vi "Monitor External Variable Clock.vi"() -> ()   [LabVIEW 2026]
uses:
  <vilib>/DAQmx/read.llb/DAQmx Read (Analog 1D Wfm NChan NSamp).vi
  <vilib>/FPGAPlugInAG/PXIe-7856R/niLvFpga_Open_PXIe-7856R.vi
  <vilib>/rvi/interface/common/dynamic/niFpgaDynamicAddResources.vi
  <vilib>/Utility/error.llb/Error Cluster From Error Code.vi
  <vilib>/rvi/errors/niLvFpgaAdjustHostInterfaceError.vi
  <vilib>/FPGAPlugInAG/Dynamic/niLvFpga_Run_Dynamic.vi
  <vilib>/DAQmx/create/channels.llb/DAQmx Create Channel (AI-Voltage-Basic).vi
  <vilib>/DAQmx/configure/timing.llb/DAQmx Timing (Sample Clock).vi
  <vilib>/DAQmx/miscellaneous.llb/DAQmx Fill In Error Info.vi
  <vilib>/measure/mascope.llb/Pulse Measurements N chan.vi
  <vilib>/FPGAPlugInAG/Dynamic/niLvFpga_Close_Dynamic.vi
  <vilib>/rvi/interface/nirviOpenFPGA/nirviOpenFPGA.xnode
  FPGA Bitfiles/PulseAndClockGeneration.lvbitx
  FPGA/Pulse and Clock Generation.vi
  <vilib>/rvi/interface/nirviReadWriteControl/nirviReadWriteControl.xnode
  <vilib>/rvi/interface/nirviMethod/nirviMethod.xnode
  <vilib>/rvi/interface/nirviCloseFPGA/nirviCloseFPGA.xnode
  <vilib>/rvi/interface/Simulation/niFpgaSimulationCallBeginRW.vi
  NiFpgaLv.dll
  <vilib>/measure/NI_MAPro.lvlib
panel:
  out "Frequency Hz":dbl
  in  "stop":bool
  out "Waveform Graph":waveform(dbl)[](graph)
  out "error out":errorcluster
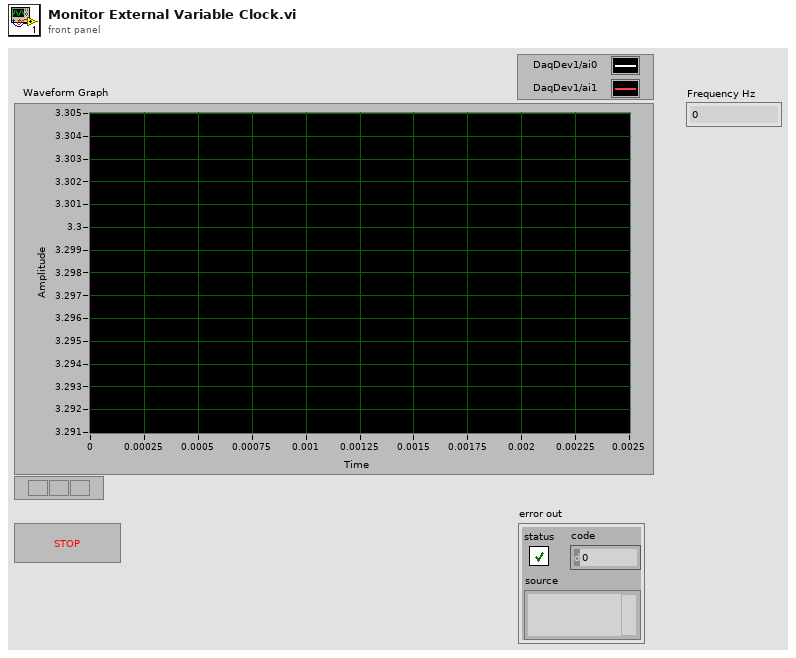
[diagram p1: front panel]
types:
  T1 = cluster{"high ref level":dbl, "mid ref level":dbl, "low ref level":dbl, "ref units":u16}
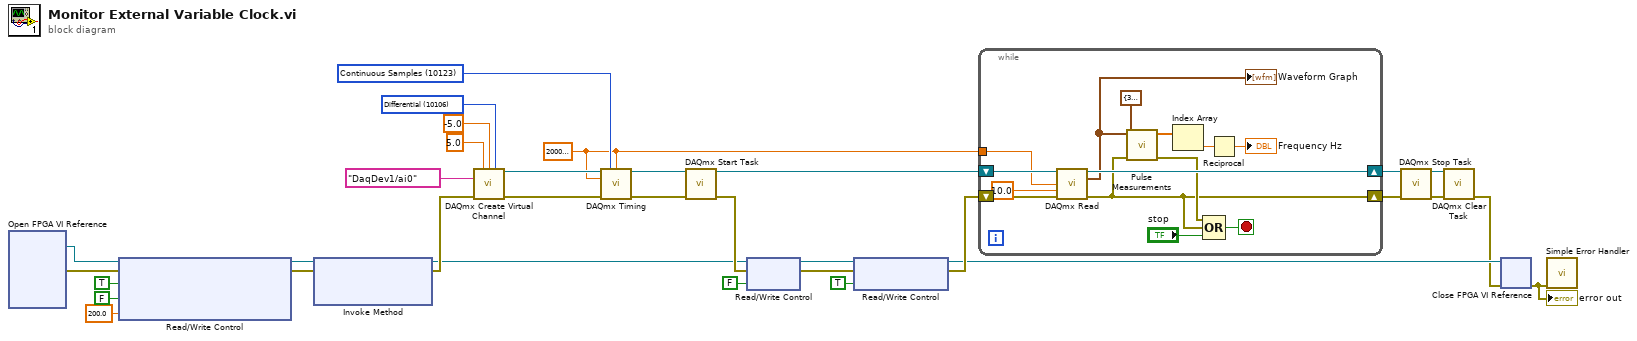
[diagram p0: block diagram]
diagram:
  w2 = 2000000.0 ("rate")
  w27 = 10123 items=["Finite Samples"=10178, "Continuous Samples"=10123, "Hardware Timed Single Point"=12522] ("sample mode")
  w32 = 10106 items=["Default"=-1, "RSE"=10083, "NRSE"=10078, "Differential"=10106, "Pseudodifferential"=12529] ("input terminal configuration")
  n1 = xnode "Open FPGA VI Reference"() -> ("FPGA VI Reference Out"=w21:refnum<k20>, "error out"=w20:errorcluster)  [unwired: 2 in]
  n2 = xnode "Read/Write Control"("FPGA VI Reference In"=w21, "error in"=w20, "Reset"=TRUE, "Enable Output"=FALSE ("Connector1/DIO0"), "Requested Output Frequency"=sgl 200.0 ("Requested Clock frequency")) -> ("FPGA VI Reference Out"=w19:refnum<k20>, "error out"=w18:errorcluster)
  n3 = xnode "Invoke Method"("FPGA VI Reference In"=w19, "error in"=w18) -> ("FPGA VI Reference Out"=w9:refnum<k20>, "error out"=w17:errorcluster)  [unwired: 1 in]
  n4 = call-poly <vilib>:"DAQmx Create Virtual Channel.vi"("maximum value"=5.0, "minimum value"=-5.0, "input terminal configuration"=w32, "physical channels"=tag "DaqDev1/ai0", "error in"=w17) -> ("task out"=w29:refnum<k21>, "error out"=w28:errorcluster)  [unwired: 9 in]
  n5 = call-poly <vilib>:"DAQmx Timing.vi"("task/channels in"=w29, "sample mode"=w27, "samples per channel"=w2, "rate"=w2, "error in"=w28) -> ("task out"=w3:refnum<k21>, "error out"=w4:errorcluster)  [unwired: 9 in]
  n6 = call <vilib>:"DAQmx Start Task.vi"("task/channels in"=w3, "error in"=w4) -> ("task out"=w26:refnum<k21>, "error out"=w10:errorcluster)  [unwired: 12 in]
  n7 = xnode "Read/Write Control"("FPGA VI Reference In"=w9, "error in"=w10, "Reset"=FALSE ("Trigger")) -> ("FPGA VI Reference Out"=w8:refnum<k20>, "error out"=w6:errorcluster)
  n8 = xnode "Read/Write Control"("FPGA VI Reference In"=w8, "error in"=w6, "Enable Output"=TRUE ("Connector1/DIO0")) -> ("FPGA VI Reference Out"=w15:refnum<k20>, "error out"=w16:errorcluster)
  n9 = while {
    shift-right: [w46] -> w25
    shift-left: w26 -> [w47]
    shift-right: [w37] -> w23
    shift-left: w16 -> [w45]
    tunnel: w2 -> [w41]
    stop <- w43 stop-if-true
    n10 = call-poly <vilib>:"DAQmx Read.vi"("task/channels in"=w47, "number of samples per channel"=w41, "timeout"=10.0, "error in"=w45) -> ("task out"=w46:refnum<k21>, "data"=w40:waveform(dbl)[], "error out"=w37:errorcluster)  [unwired: 9 in]
    "Waveform Graph" <- w40
    n11 = call-poly <vilib>:"Pulse Measurements.vi"("error in (no error)"=w37, "reference levels"=T1 {"high ref level"=3.0, "mid ref level"=2.0, "low ref level"=0.5, "ref units"=0}, "signal(s) in"=w40) -> ("error out"=w38:errorcluster, "period"=w36:dbl[])  [unwired: 4 in, 3 out]
    n12 = Index Array(array=w36) -> (element=w35:dbl)  [unwired: 1 in]
    n13 = Compound Arithmetic op=OR(w38, w37, "stop") -> (w43:bool)
    n14 = Reciprocal(x=w35) -> (1/x=→"Frequency Hz":dbl)
  }
  n15 = call <vilib>:"DAQmx Stop Task.vi"("task/channels in"=w25, "error in"=w23) -> ("task out"=w24:refnum<k21>, "error out"=w22:errorcluster)  [unwired: 12 in]
  n16 = call <vilib>:"DAQmx Clear Task.vi"("task in"=w24, "error in"=w22) -> ("error out"=w14:errorcluster)  [unwired: 13 in]
  n17 = xnode "Close FPGA VI Reference"("FPGA VI Reference In"=w15, "error in"=w14) -> ("error out"=w13:errorcluster)
  "error out" <- w13
  n18 = call <vilib>:"Simple Error Handler.vi"("error in (no error)"=w13) -> ()  [unwired: 4 in, 5 out]
